vi "Microscope.SaveImageToDisk.vi"(8 "error in (no error)":errorcluster, 9 "image data":T1, 10 "folder":path, 11 "Microscope in":refnum<class "Microscope.lvclass">) -> (0 "error out":errorcluster, 2 "path out":path, 3 "Microscope out":refnum<class "Microscope.lvclass">)   [LabVIEW 2015, in "Microscope.lvclass"]
uses:
  Microscope.lvclass
  <vilib>/picture/picture.llb/imagedata.ctl
  <userlib>/_OpenG.lib/file/file.llb/Convert File Extension (Path)__ogtk.vi
  <userlib>/_OpenG.lib/file/file.llb/Strip Path - Traditional__ogtk.vi
  <userlib>/_OpenG.lib/file/file.llb/Build Path - Traditional - path__ogtk.vi
  <userlib>/_OpenG.lib/file/file.llb/Valid Path - Traditional__ogtk.vi
  <userlib>/_OpenG.lib/file/file.llb/File Exists - Scalar__ogtk.vi
  <userlib>/_OpenG.lib/file/file.llb/Build Path - Traditional__ogtk.vi
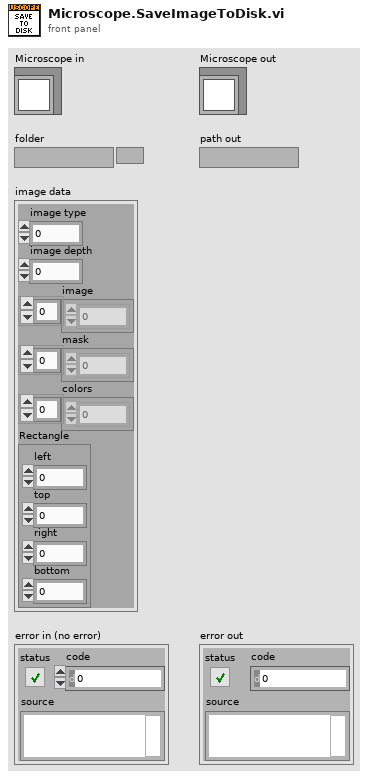
[diagram p1: front panel]
types:
  T1 = typedef "imagedata.ctl" = cluster{"image type":i32, "image depth":i32, "image":u8[], "mask":u8[], "colors":u32[], "Rectangle":cluster{"left":i16, "top":i16, "right":i16, "bottom":i16}}
  T2 = typedef "Microscope.lvclass/Configuration--Cluster.ctl" = cluster{"XY Stage":string, "Camera":string, "image output folder":path, "filetype":string}
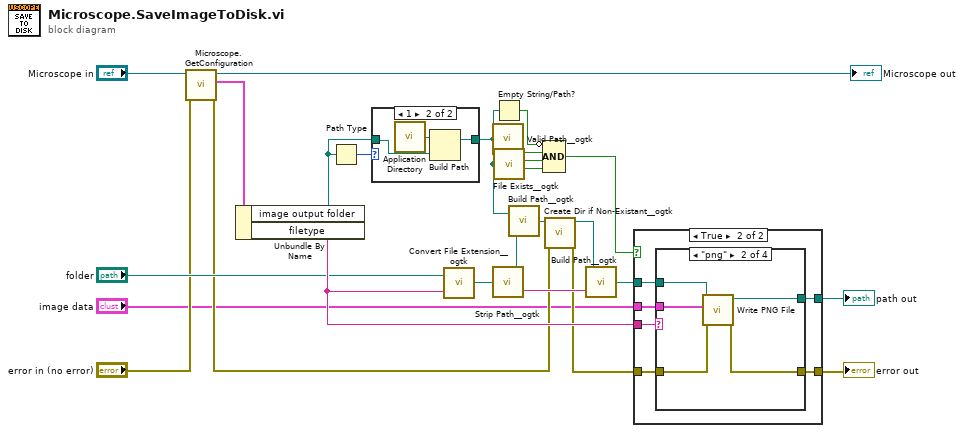
[diagram p0: block diagram]
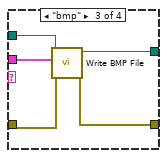
[diagram p4: hidden frame]
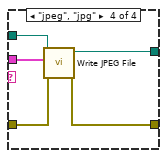
[diagram p5: hidden frame]
diagram:
  n1 = call "Microscope.GetConfiguration.vi"("error in (no error)"="error in (no error)", "Microscope"="Microscope in") -> ("error out"=w9:errorcluster, "Configuration"=w7:T2, "Microscope out"=→"Microscope out":refnum<class "Microscope.lvclass">)  [unwired: 7 in]
  n2 = Unbundle By Name(w7) -> ("image output folder"=w22:path, "filetype"=w21:string)
  n3 = Path Type(1:w22) -> (0:w14:i16)
  n4 = case shown="1" w14 {
    tunnel: w22 -> [w26 w27]
    tunnel: [w26 w29] -> w23
    frame 0, Default {
    }
    frame 1 {
      n5 = call <vilib>:"Application Directory.vi"() -> ("Application Directory"=w28:path)
      n6 = Build Path(base path=w28, name or relative path=w27) -> (appended path=w29:path)
    }
  }
  n7 = call-poly <userlib>:"Convert File Extension__ogtk.vi"("new ending (none)"=w21, "file name"="folder") -> ("new filename"=w16:path)  [unwired: 1 out]
  n8 = call-poly <userlib>:"Valid Path__ogtk.vi"("path"=w23) -> ("valid"=w12:bool)
  n9 = call-poly <userlib>:"Strip Path__ogtk.vi"("path"=w16) -> ("stripped path"=w17:path, "name"=w20:string)
  n10 = Empty String/Path?(string/path=w23) -> (empty?=w13:bool)
  n11 = call-poly <userlib>:"File Exists__ogtk.vi"("file path"=w23) -> ("is directory"=w11:bool, "exists"=w10:bool)  [unwired: 6 in]
  n12 = call-poly <userlib>:"Build Path__ogtk.vi"("name or relative path"=w17, "base path"=w23) -> ("appended path"=w18:path)
  n13 = Compound Arithmetic op=AND(invert w13, w12, w11, w10) -> (w24:bool)
  n14 = call <userlib>:"Create Dir if Non-Existant__ogtk.vi"("error in (no error)"=w9, "Directory Path"=w18) -> ("error out"=w5:errorcluster, "dup Directory Path"=w19:path)  [unwired: 7 in, 1 out]
  n15 = call-poly <userlib>:"Build Path__ogtk.vi"("name or relative path"=w20, "base path"=w19) -> ("appended path"=w4:path)
  n16 = case shown="True" w24 {
    tunnel: "image data" -> [_ w36]
    tunnel: [w30 w35] -> w3
    tunnel: w4 -> [_ w34]
    tunnel: w5 -> [w30 w33]
    tunnel: w21 -> [_ w32]
    tunnel: [_ w31] -> w25
    frame False {
    }
    frame True {
      n17 = case shown="\"png\"" w32 {
        tunnel: w36 -> [_ w42 w46 w52]
        tunnel: [w37 w41 w44 w49] -> w35
        tunnel: w34 -> [_ w40 w47 w51]
        tunnel: w33 -> [w37 w39 w45 w50]
        tunnel: [_ w38 w43 w48] -> w31
        frame Default {
        }
        frame "png" {
          n18 = call <vilib>:"Write PNG File.vi"("error in (no error)"=w39, "image data"=w42, "path to PNG file"=w40) -> ("error out"=w41:errorcluster, "path"=w38:path)  [unwired: 7 in]
        }
        frame "bmp" {
          n19 = call <vilib>:"Write BMP File.vi"("error in (no error)"=w45, "image data"=w46, "path to BMP file"=w47) -> ("error out"=w44:errorcluster, "path"=w43:path)  [unwired: 7 in]
        }
        frame "jpeg", "jpg" {
          n20 = call <vilib>:"Write JPEG File.vi"("error in (no error)"=w50, "image data"=w52, "path to JPEG file"=w51) -> ("error out"=w49:errorcluster, "path"=w48:path)  [unwired: 7 in]
        }
      }
    }
  }
  "path out" <- w25
  "error out" <- w3
